vi "Run Host.vi"(2 "Host_addon":string="_Ref") -> ()   [LabVIEW 2009, in "MoAgSy.lvlib"]
doc: "Main VI\nSets up a host system and provides functionality for local administration.\n\nHost provides a threadpool to which it deploys engine tasks for incoming agents and a separated threadpool for one dsc monitor and one dsc manager task for communication purposes\n\nAdministration:\nWhitelist to allow agent libraries, view and kill running agents by ID, show dsc monitors registered variables"
uses:
  MoAgSy.lvlib
  HGF_BaseClasses/HGF_NetworkVisitor/HGF_NetworkVisitor.lvclass
  HGF_BaseClasses/HGF_TriggeredEvent/HGF_TriggeredEvent.lvclass
  HGF_BaseClasses/HGF_Event/HGF_Event.lvclass
  MoAgSy_Engine/MoAgSy_Engine.lvclass
  HGF_BaseClasses/HGF_Reference/HGF_Reference.lvclass
  MoAgSy_Host/MoAgSy_Host.lvclass
  MoAgSy_Message/MoAgSy_Message.lvclass
  HGF_BaseClasses/HGF_ThreadPool/HGF_ThreadPool.lvclass
  HGF_BaseClasses/HGF_Factory/HGF_Factory.lvclass
panel:
  out "incoming Agents":i32
  out "incoming Messages":i32
  out "incoming NWVisitors":i32
  out "position passed":bool
  in  "stop":bool
  out "first error position":i32
  out "DSC Error":bool
  out "Incoming String":string
  out "TEST_addressee":string
  out "TEST_receiver":T1(ring)
  out "TEST_Message(s)?":bool
  in  "timeout in ms (-1)":i32=100
  in  "Application Tab":enum32{"Status", "DSC Status", "Settings"}(tab)
  out "Default Destination timed out?":bool
  out "nofTasksInQueueOut":i32
  out "nofTasksWaiting":i32
  out "autoIncrementLimit":i32=-1
  out "nofThreads":i32
  in  "Online":bool
  out "Running Agents":string[](array[string])
  out "#Running Agents":i32
  in  "killAgent":bool
  out "Host running":bool
  out "HostMonitor timed out?":bool
  out "AgentMonitor timed out?":bool
  out "Host Variable registered?":bool
  out "DSC Exception":errorcluster
  out "DSC initialNofThreads":i32
  out "DSC nofTasksWaiting":i32
  out "DSC nofThreads":i32
  out "Reg Array":T2(array[cluster])
  in  "Settings Tab":T3(tab)
  in  "Change FTP Settings":bool
  out "remote port":u16
  out "FTP Host":string
  out "FTP Username":string
  out "FTP Password":string
  out "Load new libs from FTP server":bool
  in  "Change Directories":bool
  out "Working Folder":path
  out "Class Folder":path
  out "Host Name":string
  in  "Change General Settings":bool
  out "Maximum number of running Agents":i16
  out "ID":string
  out "Library Blacklist":string[](array[string])
  in  "edit blacklist":bool
  out "Library Whitelist":string[](array[string])
  in  "edit whitelist":bool
  # "TEST"
  # "DSC Event Status (Host reachable via DSC)"
  # "ThreadPool"
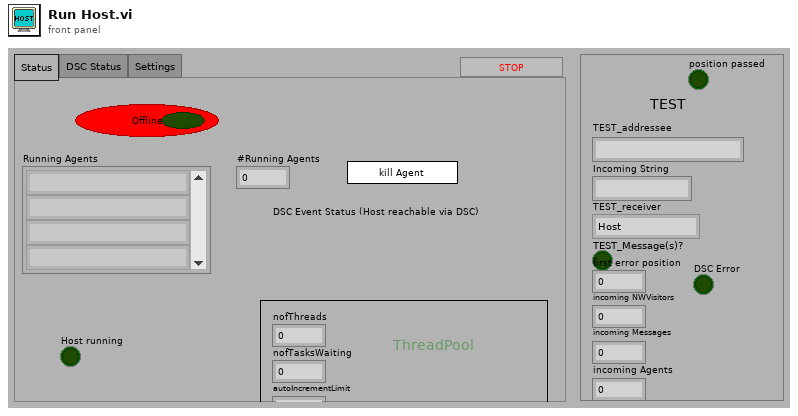
[diagram p1: front panel]
types:
  T1 = enum16{"Host", "running agent", "past Agent", "unknown"}
  T2 = cluster{"URL":string, "registered Visitors":cluster{"HGF_NetworkVisitor":refnum<class "HGF_NetworkVisitor.lvclass">, "HGF_TriggeredEvent":refnum<class "HGF_TriggeredEvent.lvclass">}[]}[]
  T3 = enum32{"FTP Settings", "Directories", "General Settings", "Blacklist", "Whitelist"}
  T4 = enum16{"Not a visitable", "Agent blacklisted", "Host full", "ok"}
  T5 = cluster{"Host Name":string, "Maximum number of running Agents":i16, "ID":string}
  T6 = cluster{"FTP Host":string, "FTP Username":string, "FTP Password":string, "remote port (21)":u16, "Load new libs from FTP server":bool}
  T7 = cluster{"Working Folder":path, "Class Folder":path}
  T8 = cluster{"DSC Event":refnum<class "HGF_Event.lvclass">}
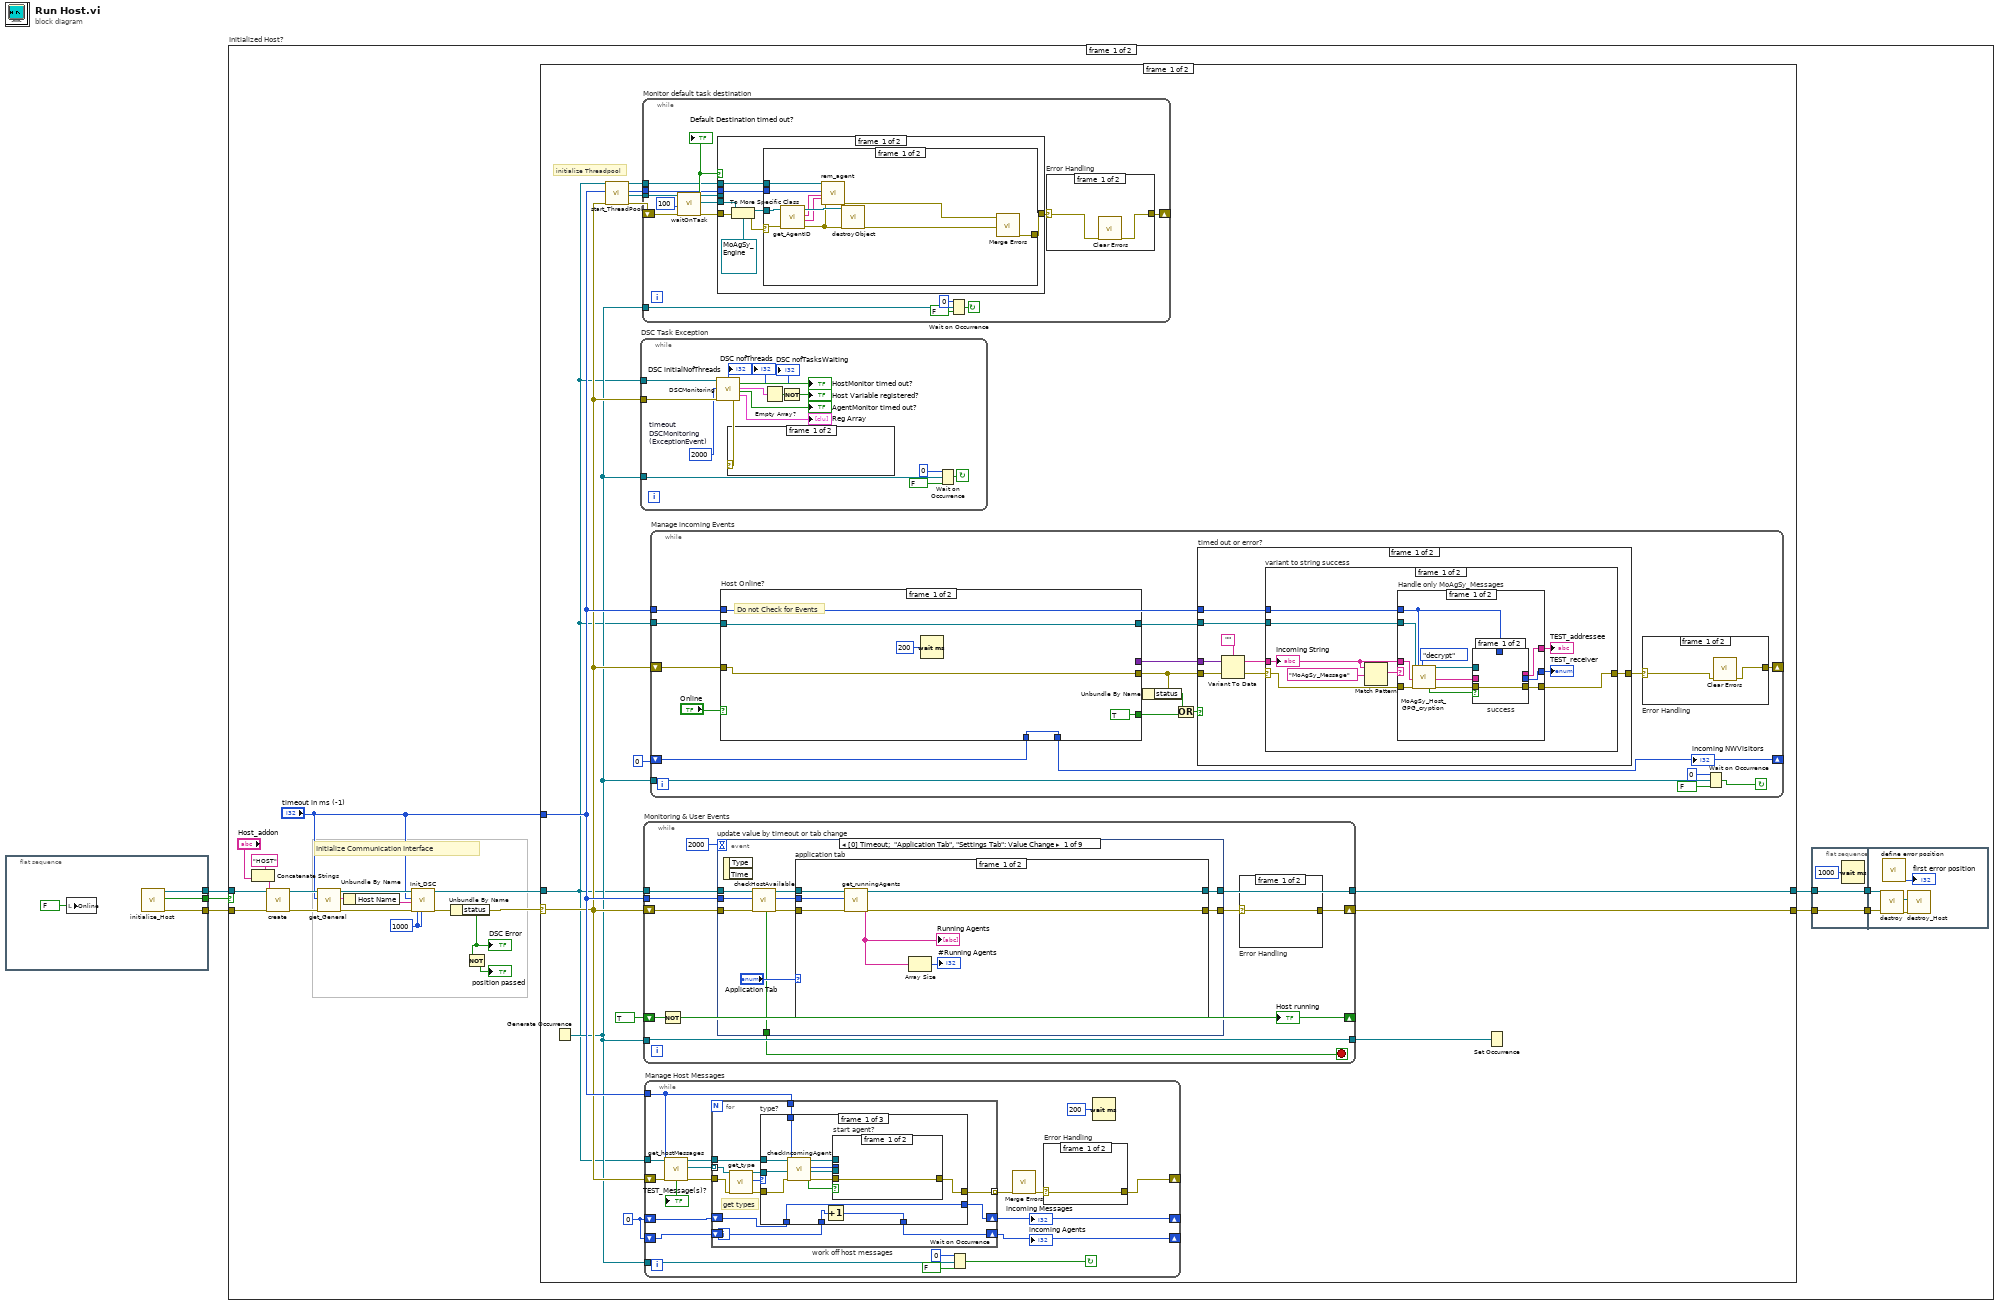
[diagram p0: block diagram]
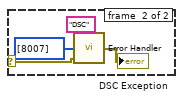
[diagram p2: hidden frame]
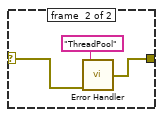
[diagram p3: hidden frame]
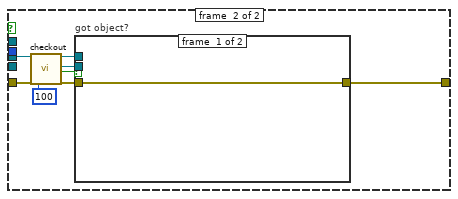
[diagram p5: hidden frame]
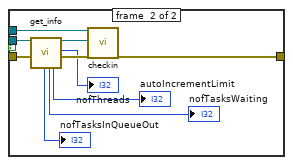
[diagram p6: hidden frame]
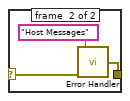
[diagram p7: hidden frame]
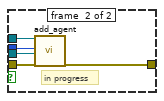
[diagram p8: hidden frame]
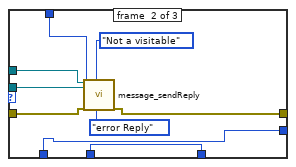
[diagram p9: hidden frame]
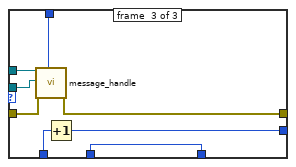
[diagram p10: hidden frame]
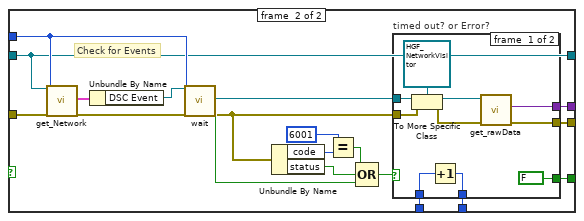
[diagram p11: hidden frame]
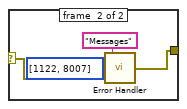
[diagram p13: hidden frame]
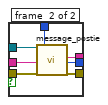
[diagram p14: hidden frame]
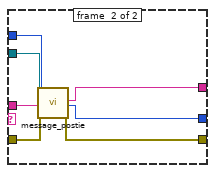
[diagram p15: hidden frame]
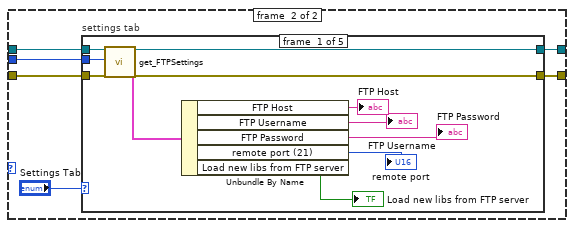
[diagram p18: hidden frame]
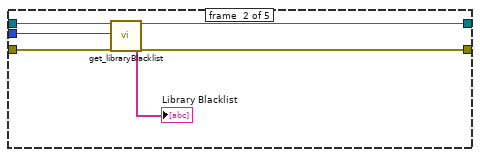
[diagram p19: hidden frame]
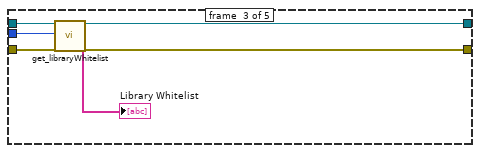
[diagram p20: hidden frame]
diagram:
  n1 = flat-sequence {
    tunnel: [w7] -> w3
    tunnel: [w4] -> w2
    tunnel: [w6] -> w1
    frame #0 {
      n2 = local write "Online"(FALSE ("Online")) -> ()
      n3 = call "initialize_Host.vi"() -> ("MoAgSy_Host out"=w7:refnum<class "MoAgSy_Host.lvclass">, "Canceled"=w6:bool, "error out"=w4:errorcluster)  [unwired: 1 in, 16 out]
    }
  }
  n4 = case "Initialized Host?" shown="False" w1 {
    tunnel: w3 -> [w28 _]
    tunnel: w2 -> [w13 _]
    frame #0 {
      w16 = 1000 ("y")
      # "Initialize Communication Interface"
      n5 = Concatenate Strings("HOST" ("name"), "Host_addon") -> (w20:string)
      n6 = call "create.vi"("Object"=w28, "name"=w20, "error in (no error)"=w13) -> ("HGF_Reference"=w19:refnum<class "HGF_Reference.lvclass">, "error out"=w11:errorcluster)  [unwired: 15 out]
      n7 = call "get_General.vi"("Host_Reference"=w19, "timeout in ms (-1)"="timeout in ms (-1)", "error in (no error)"=w11) -> ("dup Host_Reference"=w17:refnum<class "HGF_Reference.lvclass">, "General"=w27:T5, "error out"=w12:errorcluster)  [unwired: 14 out]
      n8 = Unbundle By Name(w27) -> ("Host Name"=w14:string)
      n9 = call "Init_DSC.vi"("Host_Reference"=w17, "timeout in ms (-1)"="timeout in ms (-1)", "Host Variable name"=w14, "error in (no error)"=w12, "Host Monitor timeout"=w16, "Agent Monitor timeout"=w16) -> ("dup Host_Reference"=w18:refnum<class "HGF_Reference.lvclass">, "error out"=w10:errorcluster)  [unwired: 3 in, 9 out]
      n10 = Unbundle By Name(w10) -> ("status"=w9:bool)
      "DSC Error" <- w9
      n11 = Not(x=w9) -> (.not. x?=→"position passed":bool)
      n12 = case shown="No Error" w10 {
        selector: w10 -> [w33 w434]
        tunnel: [w42 w435] -> w26
        tunnel: [w41 w434] -> w24
        tunnel: w18 -> [w31 w435]
        tunnel: "timeout in ms (-1)" -> [w35 _]
        frame #0 {
          w29 = 0
          # "initialize Threadpool"
          n13 = Generate Occurrence() -> (w32:refnum<k4>)
          n14 = call "start_ThreadPool.vi"("Host_Reference"=w31, "timeout in ms (-1)"=w35, "error in (no error)"=w33) -> ("dup Host_Reference"=w37:refnum<class "HGF_Reference.lvclass">, "dup timeout in ms"=w36:i32, "HGF_ThreadPool_Reference"=w38:refnum<class "HGF_Reference.lvclass">, "error out"=w39:errorcluster)  [unwired: 13 out]
          n15 = while "DSC Task Exception" {
            tunnel: w31 -> [w59]
            tunnel: w33 -> [w58]
            tunnel: w32 -> [w52]
            stop <- w51 continue-if-true
            w57 = 2000  # timeout DSCMonitoring (ExceptionEvent)
            n16 = call "DSCMonitoring.vi"("Host_Reference"=w59, "timeout in ms (-1)"=w57, "error in (no error)"=w58) -> ("initialNofThreads"=→"DSC initialNofThreads":i32, "nofThreads"=→"DSC nofThreads":i32, "nofTasksWaiting"=→"DSC nofTasksWaiting":i32, "DSC Exception"=w44:errorcluster, "Host timed out?"=→"HostMonitor timed out?":bool, "Registration Array"=w50:T2, "Agent timed out?"=→"AgentMonitor timed out?":bool, "Reg Array"=→"Reg Array":T2)  [unwired: 7 in, 2 out]
            n17 = case shown="Error" w44 {
              selector: w44 -> [_ w61]
              frame #0 {
              }
              frame #1 {
                n18 = call "Error Handler.vi"("error In"=w61, "ignore codes Array"=i32[] [8007] ("Array"), "key"="DSC") -> ("error Out"=→"DSC Exception":errorcluster)
              }
            }
            n19 = Empty Array?(array=w50) -> (empty?=w49:bool)
            n20 = Not(x=w49) -> (.not. x?=→"Host Variable registered?":bool)
            n21 = Wait on Occurrence(1:FALSE ("ignore previous (T)"), 2:w52, 3:0 ("ms timeout (-1)")) -> (0:w51:bool)
          }
          n22 = while "Monitor default task destination" {
            tunnel: w38 -> [w74]
            tunnel: w32 -> [w68]
            tunnel: w37 -> [w67]
            tunnel: w36 -> [w66]
            shift-right: [w64] -> _
            shift-left: w39 -> [w73]
            stop <- w69 continue-if-true
            n23 = call "waitOnTask.vi"("HGF_ThreadPool_Reference"=w74, "timeout in ms (-1)"=100, "error in (no error)"=w73) -> ("dup HGF_ThreadPool_Reference"=w78:refnum<class "HGF_Reference.lvclass">, "HGF_Task"=w76:refnum<class "HGF_ThreadTask.lvclass">, "timed out?"=w77:bool, "error out"=w72:errorcluster)  [unwired: 13 out]
            "Default Destination timed out?" <- w77
            n24 = case "timed out?" shown="False" w77 {
              tunnel: w76 -> [w91 _]
              tunnel: w72 -> [w90 w105]
              tunnel: w78 -> [_ w106]
              tunnel: w67 -> [w87 _]
              tunnel: w66 -> [w86 _]
              tunnel: [w85 w104] -> w65
              frame #0 {
                n25 = To More Specific Class(target class=refnum<class "MoAgSy_Engine.lvclass"> refnum ("MoAgSy.lvlib:MoAgSy_Engine.lvclass"), reference=w91, error in=w90) -> (specific class reference=w89:refnum<class "MoAgSy_Engine.lvclass">, error out=w88:errorcluster)
                n26 = case shown="No Error" w88 {
                  selector: w88 -> [w100 w103]
                  tunnel: w89 -> [w101 _]
                  tunnel: w87 -> [w98 _]
                  tunnel: w86 -> [w97 _]
                  tunnel: [w102 w103] -> w85
                  frame #0 {
                    n27 = call "get_AgentID.vi"("error in (no error)"=w100, "MoAgSy_Engine.lvclass in"=w101) -> ("error out"=w94:errorcluster, "destination"=w95:string, "Agent ID"=w96:string, "MoAgSy_Engine.lvclass out"=w99:refnum<class "MoAgSy_Engine.lvclass">)  [unwired: 6 out]
                    n28 = call "rem_agent.vi"("Host_Reference"=w98, "timeout in ms (-1)"=w97, "ID"=w96, "Destination"=w95, "error in (no error)"=w94) -> ("error out"=w93:errorcluster)  [unwired: 14 out]
                    n29 = call "destroyObject.vi"("HGF_Factory"=w99, "error in (no error)"=w94) -> ("error out"=w92:errorcluster)  [unwired: 17 out]
                    n30 = call <vilib>:"Merge Errors.vi"("error in 3 (no error)"=w92, "error in 1 (no error)"=w93) -> ("error out"=w102:errorcluster)  [unwired: 2 in, 3 out]
                  }
                  frame #1 {
                  }
                }
              }
              frame #1 {
                n31 = call "checkout.vi"("HGF_ThreadPool_Reference"=w106, "timeout in ms (-1)"=100, "error in (no error)"=w105) -> ("dup HGF_ThreadPool_Reference"=w107:refnum<class "HGF_Reference.lvclass">, "HGF_ThreadPool"=w108:refnum<class "HGF_ThreadPool.lvclass">, "got object?"=w111:bool, "error out"=w109:errorcluster)  [unwired: 13 out]
                n32 = case "got object?" shown="True" w111 {
                  tunnel: w107 -> [_ w122]
                  tunnel: w108 -> [_ w121]
                  tunnel: w109 -> [w112 w120]
                  tunnel: [w112 w113] -> w104
                  frame #0 {
                  }
                  frame #1 {
                    n33 = call "get_info.vi"("HGF_ThreadPool"=w121, "error in (no error)"=w120) -> ("nofTasksInQueueOut"=→"nofTasksInQueueOut":i32, "nofTasksWaiting"=→"nofTasksWaiting":i32, "autoIncrementLimit"=→"autoIncrementLimit":i32, "dup HGF_ThreadPool"=w118:refnum<class "HGF_ThreadPool.lvclass">, "nofThreads"=→"nofThreads":i32, "error out"=w119:errorcluster)  [unwired: 12 out]
                    n34 = call "checkin.vi"("HGF_Reference"=w122, "Object"=w118, "error in (no error)"=w119) -> ("error out"=w113:errorcluster)  [unwired: 1 in, 15 out]
                  }
                }
              }
            }
            n35 = Wait on Occurrence(1:FALSE ("ignore previous (T)"), 2:w68, 3:0 ("ms timeout (-1)")) -> (0:w69:bool)
            n36 = case "Error Handling" shown="Error" w65 {
              selector: w65 -> [w80 w82]
              tunnel: [w79 w83] -> w64
              frame #0 {
                n37 = call <vilib>:"Clear Errors.vi"("error in (no error)"=w80) -> ("error out"=w79:errorcluster)  [unwired: 6 out]
              }
              frame #1 {
                n38 = call "Error Handler.vi"("error In"=w82, "key"="ThreadPool") -> ("error Out"=w83:errorcluster)  [unwired: 1 in]
              }
            }
          }
          n39 = while "Monitoring & User Events" {
            tunnel: w31 -> [w311]
            tunnel: [w310] -> w42
            tunnel: w35 -> [w309]
            shift-right: [w306] -> w41
            shift-left: w33 -> [w308]
            tunnel: w32 -> [w304]
            tunnel: [w304] -> w40
            shift-right: [w301] -> _
            shift-left: TRUE -> [w302]
            stop <- w303 stop-if-true
            n40 = Not(x=w302) -> (.not. x?=w301:bool)
            "Host running" <- w301
            n41 = event "update value by timeout or tab change" shown="[0] Timeout;  \"Application Tab\", \"Settings Tab\": Value Change" {
              selector: _ -> [_ _ _ _ _ _ _ _ _]
              dyn-events: _ -> [_ _ _ _ _ _ _ _ _]
              timeout: 2000 ("Numeric") -> [_ _ _ _ _ _ _ _ _]
              tunnel: w311 -> [w318 w379 w385 w391 w397 w403 w409 w416 w429]
              tunnel: [w321 w378 w384 w390 w393 w399 w405 w411 w429] -> w310
              tunnel: w309 -> [w316 w377 w383 w389 w396 w402 w408 w415 _]
              tunnel: w308 -> [w314 w376 w382 w388 w395 w401 w407 w414 w428]
              tunnel: [w320 w375 w381 w387 w394 w400 w406 w410 w428] -> w307
              tunnel: [w312 FALSE ("NewVal") FALSE ("Stop") FALSE ("NewVal") FALSE ("NewVal") FALSE ("NewVal") FALSE ("NewVal") FALSE ("NewVal") w427] -> w303
              event #0 {
                n42 = event-data() -> ()  [unwired: 3 out]
                n43 = call "checkHostAvailable.vi"("HGF_Reference"=w318, "timeout\n in ms (-1)"=w316, "error in (no error)"=w314) -> ("STOP"=w312:bool, "dup HGF_Reference"=w317:refnum<class "HGF_Reference.lvclass">, "dup timeout\n in ms (-1)"=w315:i32, "error out"=w313:errorcluster)  [unwired: 13 out]
                n44 = case "application tab" shown="\"Status\"" "Application Tab" {
                  tunnel: w317 -> [w326 w332]
                  tunnel: [w325 w331] -> w321
                  tunnel: w315 -> [w322 w330]
                  tunnel: w313 -> [w327 w329]
                  tunnel: [w327 w328] -> w320
                  frame #0 {
                    n45 = call "get_runningAgents.vi"("Host_Reference"=w326, "timeout in ms (-1)"=w322) -> ("dup Host_Reference"=w325:refnum<class "HGF_Reference.lvclass">, "Running Agents"=w324:string[])  [unwired: 1 in, 15 out]
                    "Running Agents" <- w324
                    n46 = Array Size(array=w324) -> (size(s)=→"#Running Agents":i32)
                  }
                  frame #1 {
                    n47 = case "settings tab" shown="\"General Settings\"" "Settings Tab" {
                      tunnel: w332 -> [w344 w350 w356 w364 w373]
                      tunnel: [w343 w349 w355 w360 w370] -> w331
                      tunnel: w330 -> [w342 w346 w354 w363 w372]
                      tunnel: w329 -> [w341 w348 w353 w362 w371]
                      tunnel: [w340 w347 w352 w361 w369] -> w328
                      frame #0 {
                        n48 = call "get_FTPSettings.vi"("Host_Reference"=w344, "timeout in ms (-1)"=w342, "error in (no error)"=w341) -> ("dup Host_Reference"=w343:refnum<class "HGF_Reference.lvclass">, "FTP Settings"=w335:T6, "error out"=w340:errorcluster)  [unwired: 14 out]
                        n49 = Unbundle By Name(w335) -> ("FTP Host"=→"FTP Host":string, "FTP Username"=→"FTP Username":string, "FTP Password"=→"FTP Password":string, "remote port (21)"=→"remote port":u16, "Load new libs from FTP server"=→"Load new libs from FTP server":bool)
                      }
                      frame #1 {
                        n50 = call "get_libraryBlacklist.vi"("Host_Reference"=w350, "timeout in ms (-1)"=w346, "error in (no error)"=w348) -> ("dup Host_Reference"=w349:refnum<class "HGF_Reference.lvclass">, "Library Blacklist"=→"Library Blacklist":string[], "error out"=w347:errorcluster)  [unwired: 14 out]
                      }
                      frame #2 {
                        n51 = call "get_libraryWhitelist.vi"("Host_Reference"=w356, "timeout in ms (-1)"=w354, "error in (no error)"=w353) -> ("dup Host_Reference"=w355:refnum<class "HGF_Reference.lvclass">, "Library Whitelist"=→"Library Whitelist":string[], "error out"=w352:errorcluster)  [unwired: 14 out]
                      }
                      frame #3 {
                        n52 = call "get_Directories.vi"("Host_Reference"=w364, "timeout in ms (-1)"=w363, "error in (no error)"=w362) -> ("dup Host_Reference"=w360:refnum<class "HGF_Reference.lvclass">, "Directories"=w359:T7, "error out"=w361:errorcluster)  [unwired: 14 out]
                        n53 = Unbundle By Name(w359) -> ("Working Folder"=→"Working Folder":path, "Class Folder"=→"Class Folder":path)
                      }
                      frame #4 {
                        n54 = call "get_General.vi"("Host_Reference"=w373, "timeout in ms (-1)"=w372, "error in (no error)"=w371) -> ("dup Host_Reference"=w370:refnum<class "HGF_Reference.lvclass">, "General"=w368:T5, "error out"=w369:errorcluster)  [unwired: 14 out]
                        n55 = Unbundle By Name(w368) -> ("Host Name"=→"Host Name":string, "Maximum number of running Agents"=→"Maximum number of running Agents":i16, "ID"=→"ID":string)
                      }
                    }
                  }
                }
              }
              event #1 {
                n56 = event-data() -> ()  [unwired: 2 out]
                n57 = call "set_FTPSettings.vi"("Host_Reference"=w379, "timeout in ms (-1)"=w377, "error in (no error)"=w376) -> ("dup Host_Reference"=w378:refnum<class "HGF_Reference.lvclass">, "error out"=w375:errorcluster)  [unwired: 15 out]
              }
              event #2 {
                n58 = event-data() -> ()  [unwired: 2 out]
                n59 = call "kill_agent.vi"("Host_Reference"=w385, "timeout in ms (-1)"=w383, "error in (no error)"=w382) -> ("dup Host_Reference"=w384:refnum<class "HGF_Reference.lvclass">, "error out"=w381:errorcluster)  [unwired: 15 out]
              }
              event #3 {
                n60 = event-data() -> ()  [unwired: 2 out]
                n61 = call "set_Directories.vi"("Host_Reference"=w391, "timeout in ms (-1)"=w389, "error in (no error)"=w388) -> ("dup Host_Reference"=w390:refnum<class "HGF_Reference.lvclass">, "error out"=w387:errorcluster)  [unwired: 15 out]
              }
              event #4 {
                n62 = event-data() -> ()  [unwired: 3 out]
                n63 = call "set_General.vi"("Host_Reference"=w397, "timeout in ms (-1)"=w396, "error in (no error)"=w395) -> ("dup Host_Reference"=w393:refnum<class "HGF_Reference.lvclass">, "error out"=w394:errorcluster)  [unwired: 15 out]
              }
              event #5 {
                n64 = event-data() -> ()  [unwired: 3 out]
                n65 = call "set_libraryBlacklist.vi"("Host_Reference"=w403, "timeout in ms (-1)"=w402, "error in (no error)"=w401) -> ("dup Host_Reference"=w399:refnum<class "HGF_Reference.lvclass">, "error out"=w400:errorcluster)  [unwired: 15 out]
              }
              event #6 {
                n66 = event-data() -> ()  [unwired: 3 out]
                n67 = call "set_libraryWhitelist.vi"("Host_Reference"=w409, "timeout in ms (-1)"=w408, "error in (no error)"=w407) -> ("dup Host_Reference"=w405:refnum<class "HGF_Reference.lvclass">, "error out"=w406:errorcluster)  [unwired: 15 out]
              }
              event #7 {
                n68 = event-data() -> ("NewVal"=w413:bool)  [unwired: 1 out]
                n69 = case "Register Event/Unregister Event" shown="True" w413 {
                  tunnel: w416 -> [w421 w424]
                  tunnel: w415 -> [w420 w425]
                  tunnel: w414 -> [w419 w426]
                  tunnel: [w418 w423] -> w410
                  tunnel: [w417 w422] -> w411
                  frame #0 {
                    n70 = call "destroy_DSCEvent.vi"("Host_Reference"=w421, "timeout in ms (-1)"=w420, "error in (no error)"=w419) -> ("dup Host_Reference"=w417:refnum<class "HGF_Reference.lvclass">, "error out"=w418:errorcluster)  [unwired: 15 out]
                  }
                  frame #1 {
                    n71 = call "create_DSCEvent.vi"("Host_Reference"=w424, "timeout in ms (-1)"=w425, "error in (no error)"=w426) -> ("dup Host_Reference"=w422:refnum<class "HGF_Reference.lvclass">, "error out"=w423:errorcluster)  [unwired: 15 out]
                  }
                }
              }
              event #8 {
                w427 = TRUE  # Stop
                n72 = event-data() -> ()  [unwired: 2 out]
              }
            }
            n73 = case "Error Handling" shown="Error" w307 {
              selector: w307 -> [w430 w432]
              tunnel: [w430 w433] -> w306
              frame #0 {
              }
              frame #1 {
                n74 = call "Error Handler.vi"("error In"=w432, "key"="User Events") -> ("error Out"=w433:errorcluster)  [unwired: 1 in]
              }
            }
          }
          n75 = while "Manage Host Messages" {
            tunnel: w31 -> [w141]
            tunnel: w35 -> [w130]
            tunnel: w32 -> [w133]
            shift-right: [w127] -> _
            shift-left: w33 -> [w140]
            shift-right: [w123] -> _
            shift-left: w29 -> [w125]
            shift-right: [w124] -> _
            shift-left: w29 -> [w126]
            stop <- w132 continue-if-true
            n76 = call "get_hostMessages.vi"("Host_Reference"=w141, "timeout in ms (-1)"=w130, "error in (no error)"=w140) -> ("dup Host_Reference"=w139:refnum<class "HGF_Reference.lvclass">, "Host Messages"=w137:refnum<class "MoAgSy_Message.lvclass">[], "Message(s)?"=→"TEST_Message(s)?":bool, "error out"=w138:errorcluster)  [unwired: 13 out]
            n77 = for "work off host messages" {
              tunnel: w139 -> [w152]
              tunnel: w138 -> [w156]
              tunnel: w137 -> [w157] mode=indexing
              tunnel: w130 -> [w151]
              tunnel: [w150] -> w129 mode=indexing
              shift-right: [w148] -> w124
              shift-left: w126 -> [w149]
              shift-right: [w146] -> w123
              shift-left: w125 -> [w147]
              # "get types"
              n78 = call "get_type.vi"("MoAgSy_Message.lvclass in"=w157, "error in (no error)"=w156) -> ("MoAgSy_Message.lvclass out"=w153:refnum<class "MoAgSy_Message.lvclass">, "type"=w155:enum16{"mobile Agent", "Visitor", "Message"}, "error out"=w154:errorcluster)  [unwired: 15 out]
              n79 = case "type?" shown="\"mobile Agent\"" w155 {
                tunnel: w154 -> [w167 w182 w190]
                tunnel: w153 -> [w168 w184 w191]
                tunnel: w152 -> [w170 w185 w193]
                tunnel: w151 -> [w169 w183 w192]
                tunnel: [w161 w181 w189] -> w150
                tunnel: w149 -> [w160 w178 w188]
                tunnel: [w160 w178 w187] -> w148
                tunnel: w147 -> [w159 w177 w186]
                tunnel: [w158 w177 w186] -> w146
                frame #0 {
                  n80 = call "checkIncomingAgent.vi"("Host_Reference"=w170, "timeout in ms (-1)"=w169, "MoAgSy_Message"=w168, "error in (no error)"=w167) -> ("dup Host_Reference"=w165:refnum<class "HGF_Reference.lvclass">, "dup timeout in ms (-1)"=w164:i32, "dup MoAgSy_Message"=w163:refnum<class "MoAgSy_Message.lvclass">, "start agent?"=w166:bool, "error out"=w162:errorcluster)  [unwired: 11 out]
                  n81 = Increment(x=w159) -> (x+1=w158:i32)
                  n82 = case "start agent?" shown="True" w166 {
                    tunnel: w165 -> [_ w176]
                    tunnel: w164 -> [_ w175]
                    tunnel: w163 -> [_ w174]
                    tunnel: w162 -> [w171 w173]
                    tunnel: [w171 w172] -> w161
                    frame #0 {
                    }
                    frame #1 {
                      # "in progress"
                      n83 = call "add_agent.vi"("Host_Reference"=w176, "timeout in ms (-1)"=w175, "MoAgSy_Message"=w174, "error in (no error)"=w173) -> ("error out"=w172:errorcluster)  [unwired: 15 out]
                    }
                  }
                }
                frame #1 {
                  n84 = call "message_sendReply.vi"("Host_Reference"=w185, "MoAgSy_Message"=w184, "timeout in ms (-1)"=w183, "error in (no error)"=w182, "message"=T4."Not a visitable", "Message Type"=enum16{"error Reply", "reply"}."error Reply") -> ("error out"=w181:errorcluster)  [unwired: 1 in, 12 out]
                }
                frame #2 {
                  n85 = call "message_handle.vi"("Host_Reference"=w193, "MoAgSy_Message"=w191, "error in (no error)"=w190, "timeout in ms (-1)"=w192) -> ("error out"=w189:errorcluster)  [unwired: 15 out]
                  n86 = Increment(x=w188) -> (x+1=w187:i32)
                }
              }
            }
            "incoming Messages" <- w124
            "incoming Agents" <- w123
            n87 = Wait on Occurrence(1:FALSE ("ignore previous (T)"), 2:w133, 3:0 ("ms timeout (-1)")) -> (0:w132:bool)
            n88 = call <vilib>:"Merge Errors.vi"("error array in"=w129) -> ("error out"=w128:errorcluster)  [unwired: 3 in, 3 out]
            n89 = case "Error Handling" shown="Error" w128 {
              selector: w128 -> [w142 w144]
              tunnel: [w142 w145] -> w127
              frame #0 {
              }
              frame #1 {
                n90 = call "Error Handler.vi"("error In"=w144, "key"="Host Messages") -> ("error Out"=w145:errorcluster)  [unwired: 1 in]
              }
            }
            n91 = Wait (ms)(milliseconds to wait=u32 200) -> ()  [unwired: 1 out]
          }
          n92 = while "Manage incoming Events" {
            tunnel: w32 -> [w210]
            shift-right: [w206] -> _
            shift-left: w33 -> [w202]
            tunnel: w35 -> [w204]
            tunnel: w31 -> [w197]
            shift-right: [w194] -> _
            shift-left: 0 -> [w195]
            stop <- w208 continue-if-true
            n93 = case "Host Online?" shown="False" "Online" {
              tunnel: w197 -> [w213 w219]
              tunnel: w204 -> [_ w222]
              tunnel: [w216 w232] -> w201
              tunnel: w202 -> [w216 w231]
              tunnel: [_ w221] -> w200
              tunnel: [TRUE w220] -> w198
              tunnel: [w213 w219] -> w196
              tunnel: w195 -> [w212 w218]
              tunnel: [w212 w217] -> w194
              frame #0 {
                # "Do not Check for Events"
                n94 = Wait (ms)(milliseconds to wait=u32 200) -> ()  [unwired: 1 out]
              }
              frame #1 {
                # "Check for Events"
                n95 = call "get_Network.vi"("Host_Reference"=w219, "timeout in ms (-1)"=w222, "error in (no error)"=w231) -> ("Network"=w235:T8, "error out"=w230:errorcluster)  [unwired: 15 out]
                n96 = Unbundle By Name(w235) -> ("DSC Event"=w234:refnum<class "HGF_Event.lvclass">)
                n97 = call-dynamic "wait.vi"("HGF_Event"=w234, "msTimeout (-1)"=w222, "error in (no error)"=w230) -> ("Object"=w233:refnum<class>, "timed out"=w228:bool, "error out"=w226:errorcluster)  [unwired: 1 in, 13 out]
                n98 = Unbundle By Name(w226) -> ("code"=w225:i32, "status"=w229:bool)
                n99 = Equal?(x=6001, y=w225) -> (x = y?=w223:bool)
                n100 = Compound Arithmetic op=OR(w223, w229, w228) -> (w227:bool)
                n101 = case "timed out? or Error?" shown="True" w227 {
                  selector: w227 -> [_ w247]
                  tunnel: w233 -> [w245 _]
                  tunnel: [w239 w248] -> w232
                  tunnel: w226 -> [w241 w248]
                  tunnel: [w240 _] -> w221
                  tunnel: [FALSE w247] -> w220
                  tunnel: w218 -> [w237 w246]
                  tunnel: [w236 w246] -> w217
                  frame #0 {
                    n102 = To More Specific Class(target class=refnum<class "HGF_NetworkVisitor.lvclass"> refnum ("HGF_BaseClasses.lvlib:HGF_NetworkVisitor.lvclass"), reference=w245, error in=w241) -> (specific class reference=w243:refnum<class "HGF_NetworkVisitor.lvclass">, error out=w242:errorcluster)
                    n103 = Increment(x=w237) -> (x+1=w236:i32)
                    n104 = call "get_rawData.vi"("error in (no error)"=w242, "HGF_NetworkData"=w243) -> ("error out"=w239:errorcluster, "rawData"=w240:variant)  [unwired: 7 in, 1 out]
                  }
                  frame #1 {
                  }
                }
              }
            }
            "incoming NWVisitors" <- w194
            n105 = Unbundle By Name(w201) -> ("status"=w199:bool)
            n106 = Or(x=w199, y=w198) -> (x .or. y?=w209:bool)
            n107 = case "timed out or error?" shown="False" w209 {
              tunnel: w200 -> [w259 _]
              tunnel: [w262 w300] -> w207
              tunnel: w201 -> [w258 w300]
              tunnel: w196 -> [w261 _]
              tunnel: w204 -> [w260 _]
              frame #0 {
                n108 = Variant To Data(error in=w258, Variant=w259, type="") -> (error out=w255:errorcluster, data=w256:string)
                n109 = case "variant to string success" shown="No Error" w255 {
                  selector: w255 -> [w265 w299]
                  tunnel: w256 -> [w268 _]
                  tunnel: [w271 w299] -> w262
                  tunnel: w261 -> [w270 _]
                  tunnel: w260 -> [w266 _]
                  frame #0 {
                    n110 = Match Pattern(string=w268, regular expression="MoAgSy_Message") -> (match substring=w269:string)  [unwired: 4 out]
                    n111 = case "Handle only MoAgSy_Messages" shown="\"MoAgSy_Message\"" w269 {
                      tunnel: w265 -> [w283 w298]
                      tunnel: [w275 w296] -> w271
                      tunnel: w270 -> [w282 w294]
                      tunnel: w268 -> [w272 w297]
                      tunnel: w266 -> [w276 w295]
                      tunnel: [w274 w293] -> w264
                      tunnel: [w273 w292] -> w263
                      frame #0 {
                        n112 = call "MoAgSy_Host_GPG_cryption.vi"("Host_Reference"=w282, "string in"=w272, "error in (no error)"=w283, "timeout in ms (-1)"=w276, "task"=enum16{"encrypt", "decrypt", "sign", "verify"}."decrypt") -> ("success"=w279:bool, "dup Host_Reference"=w277:refnum<class "HGF_Reference.lvclass">, "String out"=w278:string, "error out"=w280:errorcluster)  [unwired: 11 in]
                        n113 = case "success" shown="True" w279 {
                          tunnel: w280 -> [w284 w288]
                          tunnel: w278 -> [_ w289]
                          tunnel: w277 -> [_ w291]
                          tunnel: w276 -> [_ w290]
                          tunnel: [w284 w287] -> w275
                          tunnel: [_ w286] -> w274
                          tunnel: [_ w285] -> w273
                          frame #0 {
                          }
                          frame #1 {
                            n114 = call "message_postie.vi"("HGF_Reference"=w291, "String"=w289, "error IO"=w288, "timeout in ms (-1)"=w290) -> ("TEST_addressee"=w286:string, "TEST_receiver"=w285:T1, "error out"=w287:errorcluster)  [unwired: 13 in]
                          }
                        }
                      }
                      frame #1 {
                        n115 = call "message_postie.vi"("HGF_Reference"=w294, "String"=w297, "error IO"=w298, "timeout in ms (-1)"=w295) -> ("TEST_addressee"=w293:string, "TEST_receiver"=w292:T1, "error out"=w296:errorcluster)  [unwired: 13 in]
                      }
                    }
                    "TEST_addressee" <- w264
                    "TEST_receiver" <- w263
                    "Incoming String" <- w268
                  }
                  frame #1 {
                  }
                }
              }
              frame #1 {
              }
            }
            n116 = case "Error Handling" shown="Error" w207 {
              selector: w207 -> [w250 w253]
              tunnel: [w249 w254] -> w206
              frame #0 {
                n117 = call <vilib>:"Clear Errors.vi"("error in (no error)"=w250) -> ("error out"=w249:errorcluster)  [unwired: 6 in]
              }
              frame #1 {
                n118 = call "Error Handler.vi"("error In"=w253, "ignore codes Array"=i32[] [1122, 8007] ("Array"), "key"="Messages") -> ("error Out"=w254:errorcluster)
              }
            }
            n119 = Wait on Occurrence(1:FALSE ("ignore previous (T)"), 2:w210, 3:0 ("ms timeout (-1)")) -> (0:w208:bool)
          }
          n120 = Set Occurrence(w40) -> ()
        }
        frame #1 {
          n121 = call <vilib>:"Simple Error Handler.vi"("error in (no error)"=w434) -> ()  [unwired: 4 in, 5 out]
        }
      }
      n122 = flat-sequence {
        tunnel: w26 -> [w437]
        tunnel: [w437] -> w25
        tunnel: w24 -> [w436]
        tunnel: [w436] -> w23
        tunnel: w25 -> [w443]
        tunnel: w23 -> [w442]
        frame #0 {
          n123 = Wait (ms)(milliseconds to wait=u32 1000) -> ()  [unwired: 1 out]
        }
        frame #1 {
          n124 = call "destroy.vi"("HGF_Reference"=w443, "error in (no error)"=w442) -> ("Object"=w440:refnum<class>, "error out"=w441:errorcluster)  [unwired: 2 in, 14 out]
          n125 = call "define error position.vi"() -> ("first error position"=→"first error position":i32)  [unwired: 10 in, 1 out]
          n126 = call "destroy_Host.vi"("error in (no error)"=w441, "LabVIEW Object"=w440) -> ()  [unwired: 1 in, 9 out]
        }
      }
    }
    frame #1 {
    }
  }
